vi "Induction Range Save Data.vi"(8 "Error In":errorcluster, 9 "Data":string[][](array[string]), 10 "Save Data":bool, 11 "Choose Folder":path) -> (0 "Error Out":errorcluster)   [LabVIEW 2016]
uses:
  <vilib>/Utility/file.llb/Write Delimited Spreadsheet (string).vi
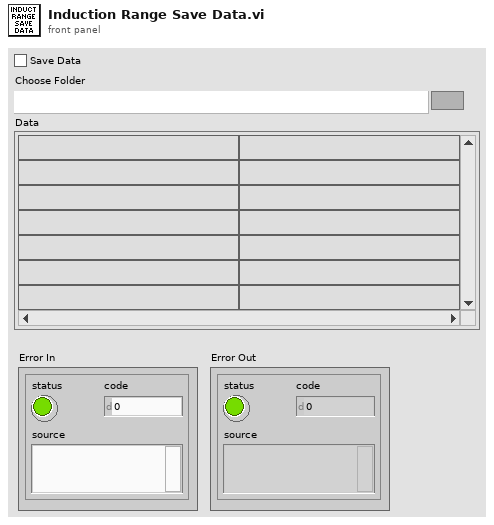
[diagram p1: front panel]
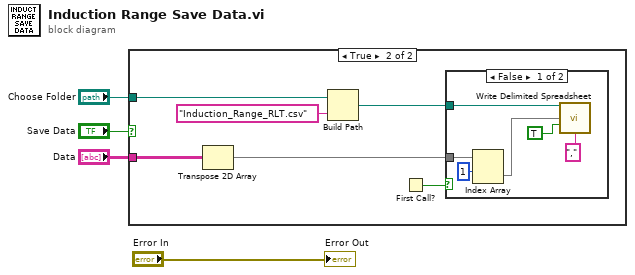
[diagram p0: block diagram]
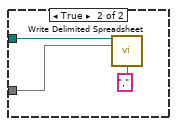
[diagram p3: hidden frame]
diagram:
  n1 = case shown="True" "Save Data" {
    tunnel: "Choose Folder" -> [_ w9]
    tunnel: "Data" -> [_ w7]
    frame False {
    }
    frame True {
      n2 = Transpose 2D Array(2D array=w7) -> (transposed array=w6:string[][])
      n3 = Build Path(base path=w9, name or relative path="Induction_Range_RLT.csv") -> (appended path=w8:path)
      n4 = First Call?() -> (First Call?: T/F=w5:bool)
      n5 = case shown="False" w5 {
        tunnel: w8 -> [w14 w19]
        tunnel: w6 -> [w16 w18]
        frame False {
          n6 = Index Array(array=w16, index (row)=1) -> (element=w13:string[])  [unwired: 1 in]
          n7 = call-poly <vilib>:"Write Delimited Spreadsheet.vi"("file path (dialog if empty)"=w14, "1D data"=w13, "append to file? (new file:F)"=TRUE, "delimiter (\\t)"="," ("delimiter (\\t)")) -> ()  [unwired: 10 in, 2 out]
        }
        frame True {
          n8 = call-poly <vilib>:"Write Delimited Spreadsheet.vi"("file path (dialog if empty)"=w19, "2D data"=w18, "delimiter (\\t)"="," ("delimiter (\\t)")) -> ()  [unwired: 11 in, 2 out]
        }
      }
    }
  }
  "Error Out" <- "Error In"
